vi "Circular Buffer (waveforms).vi"(6 "History Length [1024]":i32=1024, 7 "reset":bool, 8 "error in":errorcluster, 11 "Waveform in":waveform(dbl)[](array[waveform])) -> (0 "error out":errorcluster, 3 "Waveform out":waveform(dbl)[](array[waveform]))   [LabVIEW 2019, in "xy_utilities.lvlib"]
doc: "Circular Buffer with controllable reset and history length."
uses:
  xy_utilities.lvlib
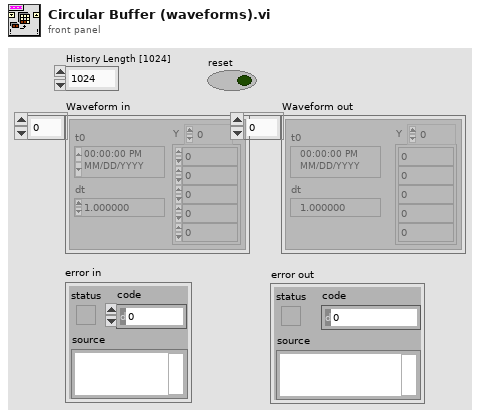
[diagram p1: front panel]
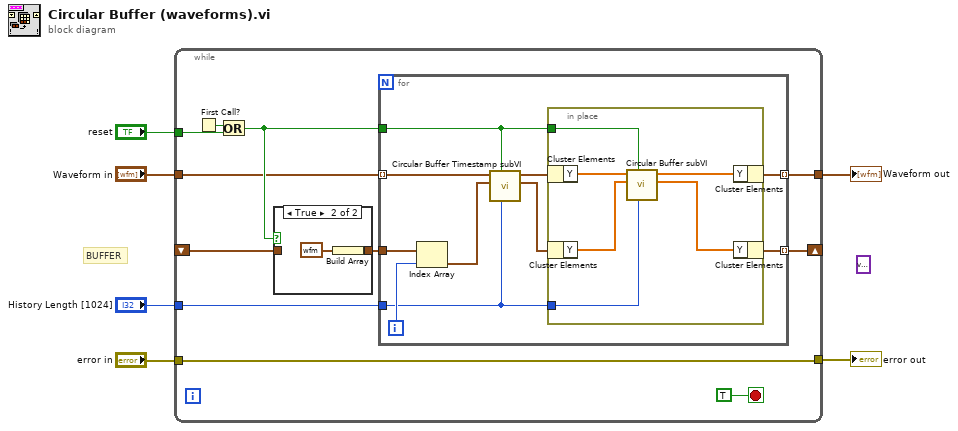
[diagram p0: block diagram]
diagram:
  (unwired) variant
  # "BUFFER"
  n1 = while {
    tunnel: "Waveform in" -> [w10]
    tunnel: [w17] -> w3
    tunnel: "error in" -> [w17]
    tunnel: "reset" -> [w15]
    shift-right: [w7] -> _
    shift-left: _ -> [w11]
    tunnel: "History Length [1024]" -> [w13]
    tunnel: [w9] -> w1
    stop <- TRUE stop-if-true
    n2 = First Call?() -> (First Call?: T/F=w16:bool)
    n3 = Or(x=w16, y=w15) -> (x .or. y?=w12:bool)
    n4 = case shown="True" w12 {
      tunnel: w11 -> [w34 _]
      tunnel: [w34 w35] -> w8
      frame False {
      }
      frame True {
        n5 = Build Array(waveform(dbl) {"t0"=timestamp(0 s since 1904-01-01), "dt"=1.0, "Y"=[]} ("Waveform in")) -> (w35:waveform(dbl)[])
      }
    }
    n6 = for {
      tunnel: w13 -> [w20]
      tunnel: w12 -> [w23]
      tunnel: w10 -> [w21] mode=indexing
      tunnel: [w27] -> w9 mode=indexing
      tunnel: w8 -> [w26]
      tunnel: [w25] -> w7 mode=indexing
      i -> [w24]
      n7 = Index Array(array=w26, index=w24) -> (element=w19:waveform(dbl))
      n8 = call "Circular Buffer Timestamp subVI.vi"("History Length [1024]"=w20, "reset"=w23, "Buffer in"=w19, "Waveform in in"=w21) -> ("Buffer out"=w18:waveform(dbl), "Waveform out"=w22:waveform(dbl))  [unwired: 6 in]
      n9 = in-place {
        in-place-border: w20 -> [w33]
        in-place-border: w23 -> [w32]
        n10 = in-place-cluster #1(w22) -> ("Y"=w31:dbl[])
        n11 = in-place-cluster #2(w18) -> ("Y"=w29:dbl[])
        n12 = call "Circular Buffer subVI.vi"("History Length [1024]"=w33, "Reset"=w32, "Buffer in"=w29, "Array in"=w31) -> ("Buffer out"=w28:dbl[], "Array out"=w30:dbl[])  [unwired: 6 in]
        n13 = in-place-cluster #1("Y"=w30) -> (w27:waveform(dbl))
        n14 = in-place-cluster #2("Y"=w28) -> (w25:waveform(dbl))
      }
    }
  }
  "Waveform out" <- w1
  "error out" <- w3
